vi "testSendCmd.vi"(8 "error in (no error)":errorcluster) -> (0 "error out":errorcluster)   [LabVIEW 2018]
panel:
  in  "iterations":i32=10
  in  "milliseconds to wait":u32=100
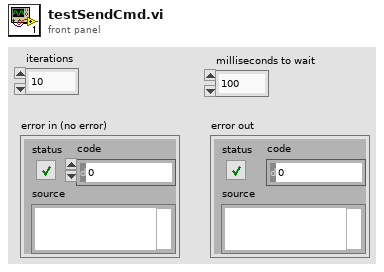
[diagram p1: front panel]
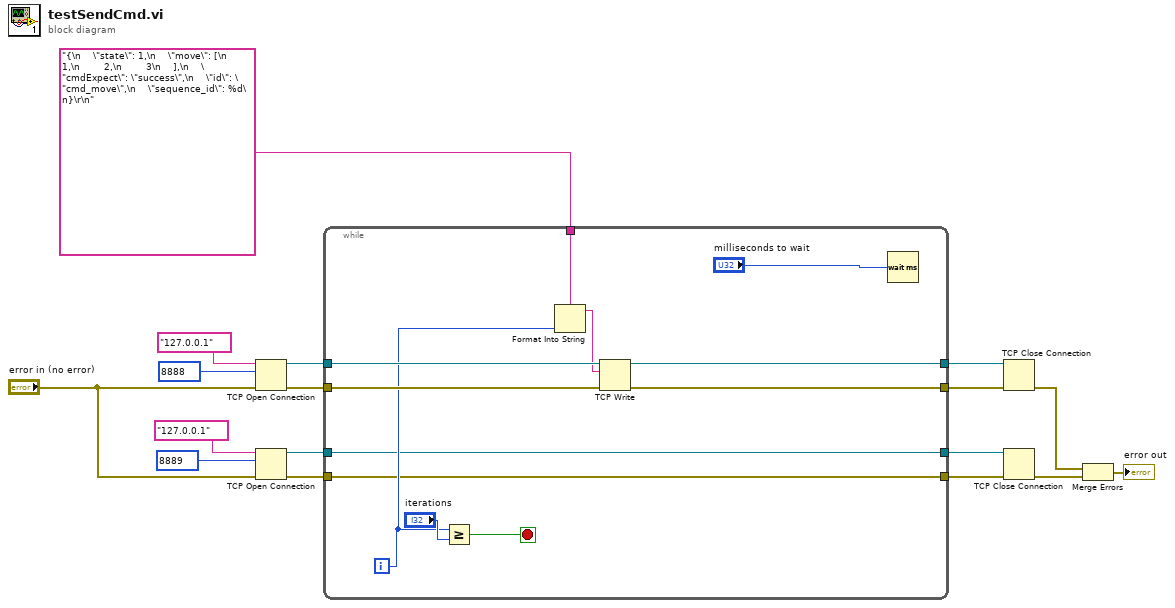
[diagram p0: block diagram]
diagram:
  n1 = TCP Open Connection(address="127.0.0.1", remote port or service name=u16 8888, error in (no error)="error in (no error)") -> (connection ID=w9:refnum<k5>, error out=w8:errorcluster)  [unwired: 2 in]
  n2 = TCP Open Connection(address="127.0.0.1", remote port or service name=u16 8889, error in (no error)="error in (no error)") -> (connection ID=w6:refnum<k5>, error out=w7:errorcluster)  [unwired: 2 in]
  n3 = while {
    tunnel: w9 -> [w29]
    tunnel: w8 -> [w28]
    tunnel: [w22] -> w4
    tunnel: [w21] -> w1
    tunnel: w7 -> [w21]
    tunnel: [w20] -> w2
    tunnel: w6 -> [w20]
    tunnel: [w19] -> w3
    tunnel: "{\n    \"state\": 1,\n    \"move\": [\n        1,\n        2,\n        3\n    ],\n    \"cmdExpect\": \"success\",\n    \"id\": \"cmd_move\",\n    \"sequence_id\": %d\n}\r\n" ("Display") -> [w18]
    i -> [w25]
    stop <- w24 stop-if-true
    n4 = Greater Or Equal?(x=w25, y="iterations") -> (x >= y?=w24:bool)
    n5 = Format Into String(format string=w18, w25) -> (resulting string=w23:string)  [unwired: 2 in, 1 out]
    n6 = TCP Write(connection ID=w29, data in=w23, error in (no error)=w28) -> (connection ID out=w22:refnum<k5>, error out=w19:errorcluster)  [unwired: 1 in, 1 out]
    n7 = Wait (ms)(milliseconds to wait="milliseconds to wait") -> ()  [unwired: 1 out]
  }
  n8 = TCP Close Connection(connection ID=w4, error in (no error)=w3) -> (error out=w15:errorcluster)  [unwired: 1 in, 1 out]
  n9 = TCP Close Connection(connection ID=w2, error in (no error)=w1) -> (error out=w14:errorcluster)  [unwired: 1 in, 1 out]
  n10 = Merge Errors(w15, w14) -> (→"error out":errorcluster)
